vi "test_Error Code Channel Waveform Incoming.vi"(8 "error in (no error)":errorcluster, 11 "TestCase in":refnum<class "DMA Waveform Status Channel Testing.lvclass">) -> (0 "error out":errorcluster, 3 "TestCase out":refnum<class "DMA Waveform Status Channel Testing.lvclass">)   [LabVIEW 2019, in "DMA Waveform Status Channel Testing.lvclass"]
uses:
  DMA Waveform Status Channel Testing.lvclass
  <vilib>/addons/_JKI Toolkits/VI Tester/TestCase.llb/TestCase.lvclass
  C:/Program Files (x86)/National Instruments/LabVIEW 2019/vi.lib/addons/_JKI Toolkits/VI Tester/TestCase.llb/TestCase.lvclass
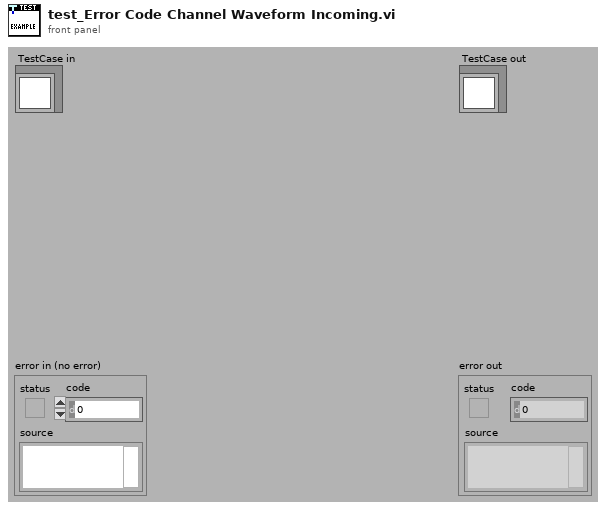
[diagram p1: front panel]
types:
  T1 = typedef "NI_VS Workspace ExecutionAPI.lvlib/WorkspaceAPI.ctl" = refnum<k24>
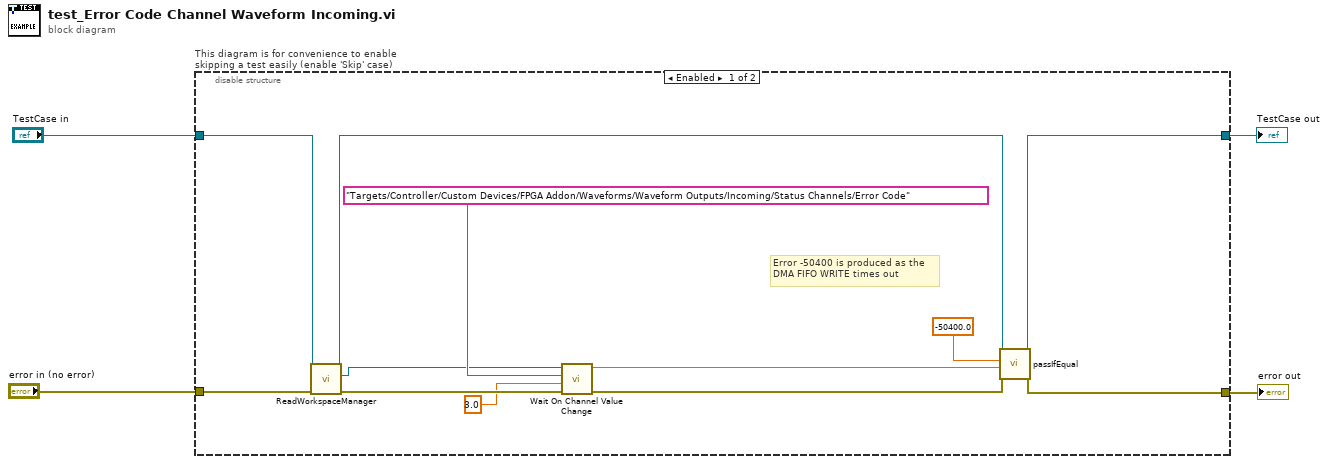
[diagram p0: block diagram]
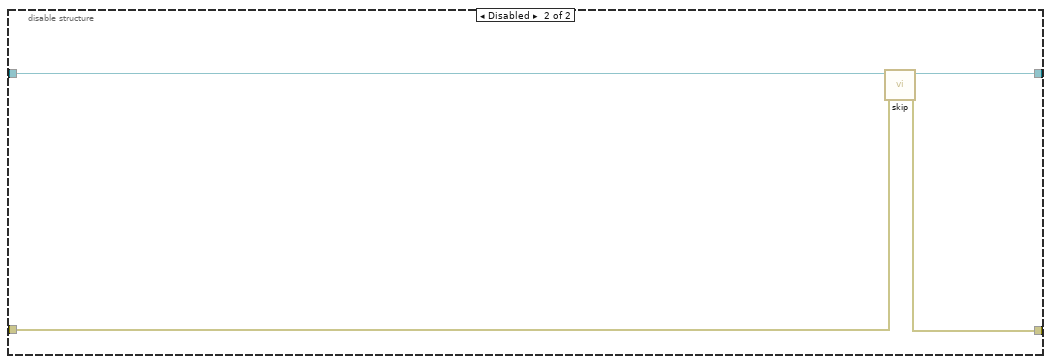
[diagram p2: hidden frame]
diagram:
  n1 = disable-structure "This diagram is for convenience to enable skipping a test easily (enable 'Skip' case)" shown="Enabled" {
    disable-tunnel: "TestCase in" -> [w11 w20]
    disable-tunnel: [w16 w18] -> w1
    disable-tunnel: [w15 w19] -> w3
    disable-tunnel: "error in (no error)" -> [w13 w17]
    frame Enabled {
      # "Error -50400 is produced as the \nDMA FIFO WRITE times out"
      n2 = call-dynamic "ReadWorkspaceManager.vi"("error in (no error)"=w13, "VeriStand Test Case in"=w11) -> ("error out"=w10:errorcluster, "Workspace"=w7:T1, "VeriStand Test Case out"=w12:refnum<class "DMA Waveform Status Channel Testing.lvclass">)  [unwired: 7 in]
      n3 = call "Wait On Channel Value Change.vi"("error in (no error)"=w10, "Time to Wait"=3.0, "Channel"="Targets/Controller/Custom Devices/FPGA Addon/Waveforms/Waveform Outputs/Incoming/Status Channels/Error Code", ".NET Refnum in"=w7) -> ("error out"=w9:errorcluster, "Value"=w6:dbl)  [unwired: 6 in]
      n4 = call-dynamic "passIfEqual.vi"("error in (no error)"=w9, "y"=w6, "x"=-50400.0 ("Value"), "TestCase in"=w12) -> ("error out"=w15:errorcluster, "TestCase out"=w16:refnum<class "DMA Waveform Status Channel Testing.lvclass">)  [unwired: 6 in]
    }
    frame Disabled {
      # "skip test result while test is under development"
      n5 = call <vilib>:"skip.vi"("error in (no error)"=w17, "TestCase in"=w20) -> ("error out"=w19:errorcluster, "TestCase out"=w18:refnum<class "DMA Waveform Status Channel Testing.lvclass">)  [unwired: 8 in]
    }
  }
  "error out" <- w3
  "TestCase out" <- w1
